vi "CSMLS - Continuous Loop in CSM Example.vi"() -> ()   [LabVIEW 2017]
uses:
  user.lib/_NEVSTOP/Communicable State Machine(CSM)/AdvanceAPI/CSM - Revert Arguments-Safe String.vi
  user.lib/_NEVSTOP/Communicable State Machine(CSM)/AdvanceAPI/CSM - Make String Arguments Safe.vi
  user.lib/_NEVSTOP/Communicable State Machine(CSM)/AdvanceAPI/CSM - Break Down Multiple States String.vi
  user.lib/_NEVSTOP/Communicable State Machine(CSM)/AdvanceAPI/CSM - Compact Multiple States.vi
  user.lib/_NEVSTOP/Communicable State Machine(CSM)/AdvanceAPI/CSM - Keywords.vi
  user.lib/_NEVSTOP/Communicable State Machine(CSM)/_Polymophic/CSM - Filter Duplicated Lines.vi
  user.lib/_NEVSTOP/Communicable State Machine(CSM)/_Shared/Trim Single-line Text.vi
  user.lib/_NEVSTOP/Communicable State Machine(CSM)/Communicable State Machine.lvlib
  user.lib/_NEVSTOP/Communicable State Machine(CSM)/addons/Loop-Support/CSM Loop Support.lvlib
  user.lib/_NEVSTOP/Communicable State Machine(CSM)/addons/Logger/CSM File Logger.lvlib
panel:
  in  "Enable Periodic State Filter(T)":bool=TRUE
  in  "High-Priority Error":bool
  in  "Low-Priority Error":bool
  out "Filtered UI States":string="Macro: DAQ Continuous"
  out "UI States":string="Macro: DAQ Continuous"
  out ">> From CSM >>":string="<loop>"
  out "Remaining States":string="Exit"
  in  "DAQ: Once":bool
  out "Waveform Chart":dbl(graph)=0.33666580363788867
  in  "Center":dbl(slide) scale=0.0..10.0
  in  "Stop":bool
  in  "Start":bool
  out "State History":string="--------------------\nPeroid State:\nFilter #17 since 00:04:42.203 - DAQ: Continuous Check >> 0.902887\rFilter #18 since 00:04:42.203 - Data: Acquisite\n--------------------\n[00:04:45.825] Exit\r[00:04:45.823] Data: Cleanup\r[00:04:45.823] Macro: Exit\r[00:04:45.818] UI: Refresh Buttons <- <end>\r[00:04:45.817] DAQ: Close\r[00:04:45.817] DAQ: Stop\r[00:04:42.203] <Start Filter>DAQ: Continuous Check\r[00:04:42.203] <Start Filter>Data: Acquisite\r[00:04:42.003] DAQ: Continuous Check >> 0.591368 <- <loop>\r[00:04:42.003] Data: Acquisite\r[00:04:41.804] DAQ: Continuous Check >> 0.572752 <- <loop>\r[00:04:41.803] Data: Acquisite\r[00:04:41.603] DAQ: Continuous Check >> 0.632503 <- <loop>\r[00:04:41.603] Data: Acquisite\r[00:04:41.403] DAQ: Continuous Check >> 0.461989 <- <loop>\r[00:04:41.402] Data: Acquisite\r[00:04:41.202] DAQ: Continuous Check <- <loop>\r[00:04:41.201] Data: Acquisite\r[00:04:41.069] UI: Refresh Buttons\r[00:04:41.069] DAQ: Start\r[00:04:41.069] DAQ: Configure\r[00:04:41.069] DAQ: Initialize\r[00:04:41.068] Macro: DAQ Continuous\r[00:04:40.593] Data: Update Indicators\r[00:04:40.588] UI: Refresh Buttons\r[00:04:40.585] UI: Initialize\r[00:04:40.584] Initialize Core Data\r[00:04:40.584] Data: Initialize\r[00:04:40.583] Macro: Initialize\r"
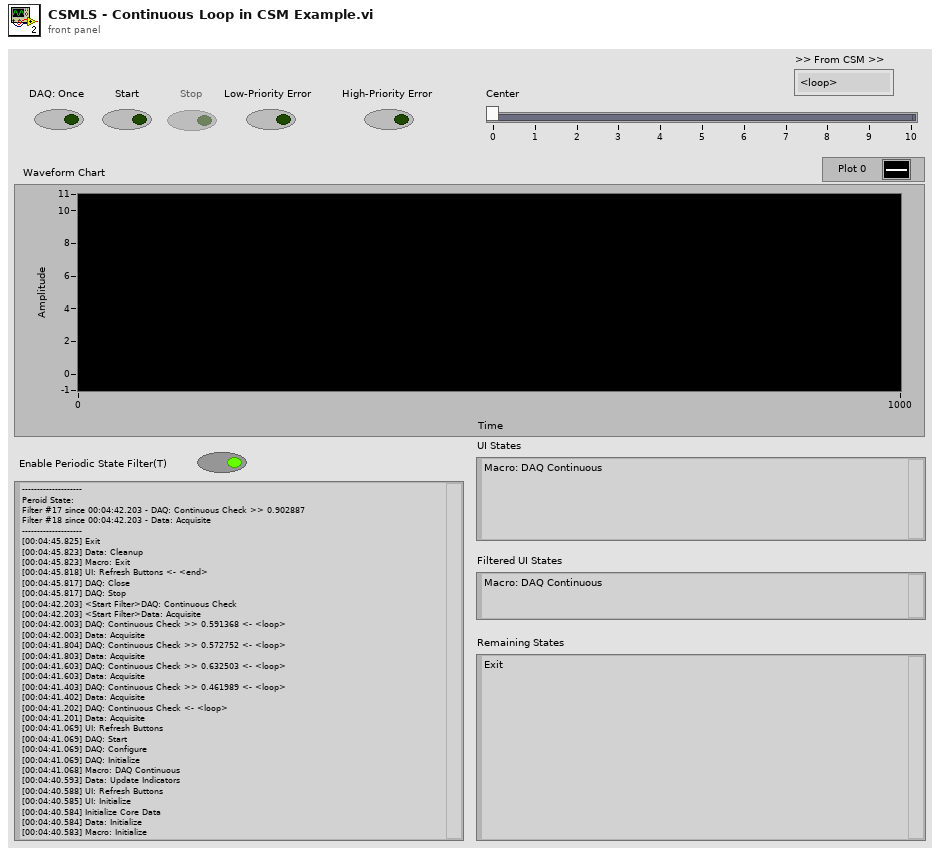
[diagram p1: front panel]
types:
  T1 = enum32{"Invalid", "Standard", "Closed", "Hidden", "Minimized", "Maximized"}
  T2 = enum32{"invalid app kind", "Development System", "Run Time System", "Student Edition", "Embedded LabVIEW", "Evaluation", "Custom"}
  T3 = typedef "Communicable State Machine.lvlib/_CSM_Response Source Message.ctl" = cluster{"‘State":string, "’Arguments":string, "’Error":errorcluster}
  T4 = cluster{"Current VI Reference":refnum<vi>, "Close Panel on Exit?":bool}
  T5 = cluster{"Core":cluster{"Current VI Reference":refnum<vi>, "Close Panel on Exit?":bool}, "IsRunning?":bool, "Center":dbl}
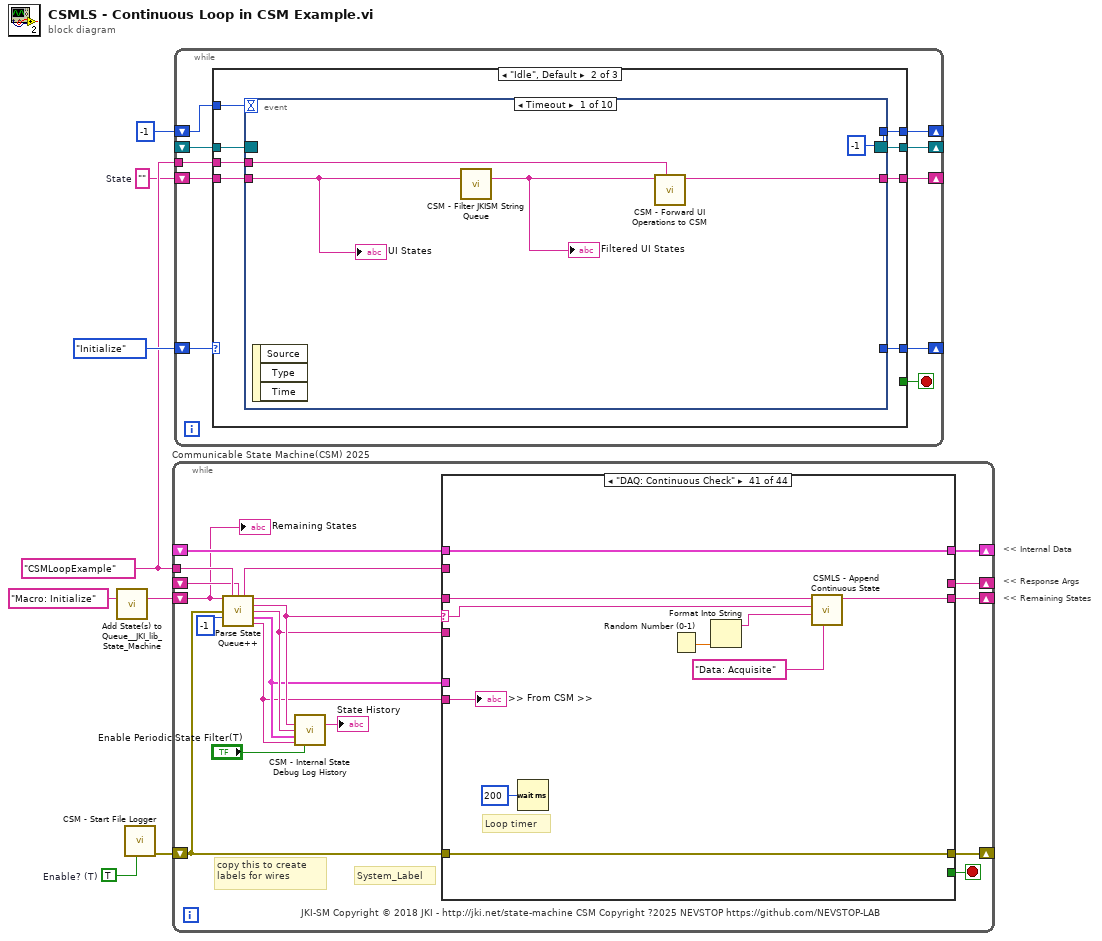
[diagram p0: block diagram]
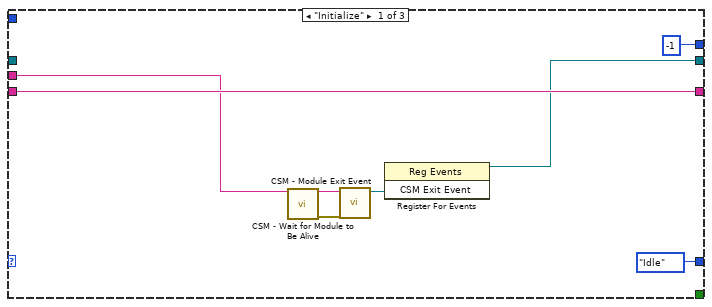
[diagram p2: hidden frame]
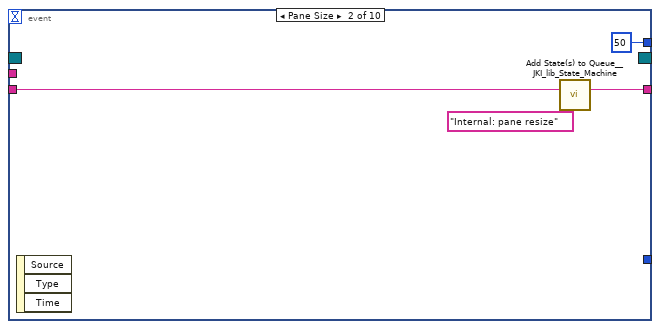
[diagram p3: hidden frame]
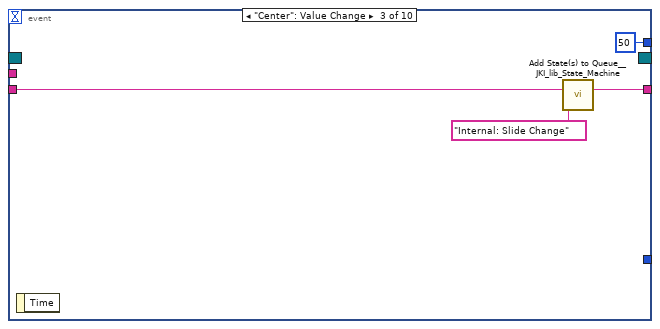
[diagram p4: hidden frame]
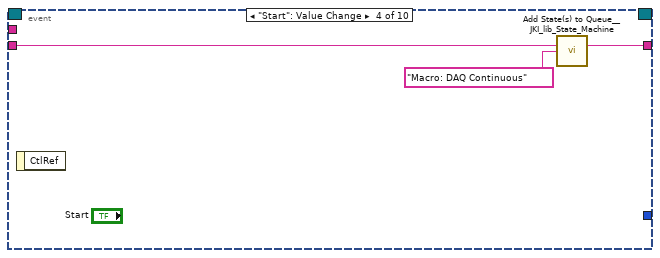
[diagram p5: hidden frame]
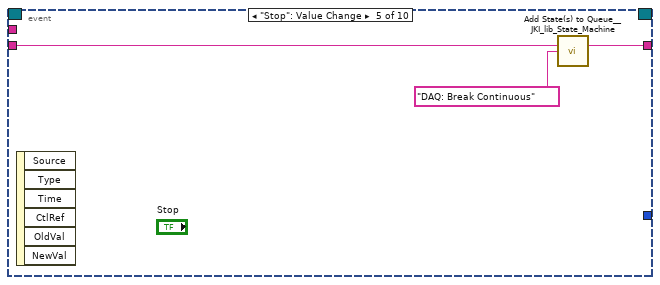
[diagram p6: hidden frame]
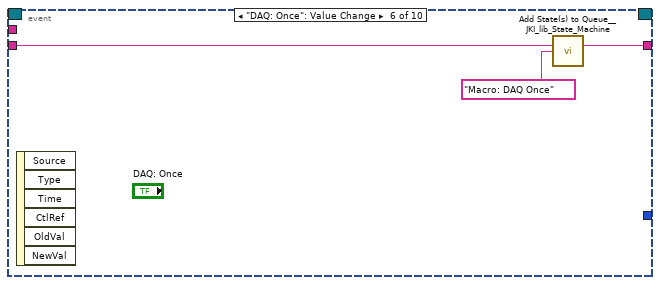
[diagram p7: hidden frame]
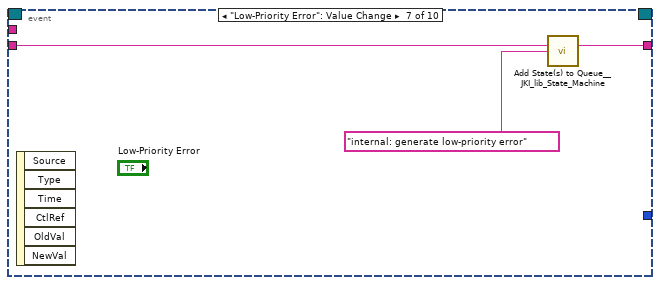
[diagram p8: hidden frame]
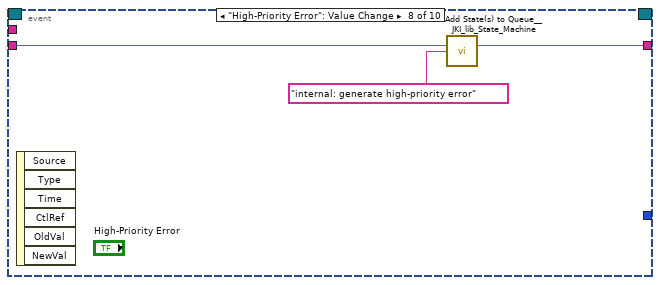
[diagram p9: hidden frame]
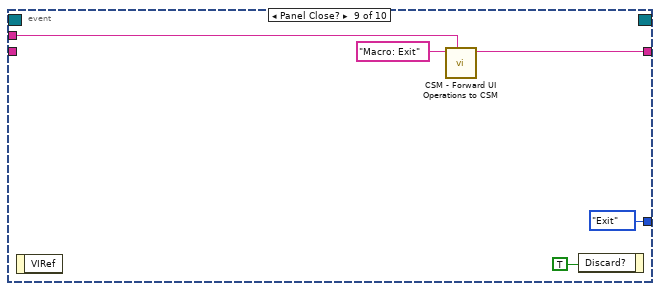
[diagram p10: hidden frame]
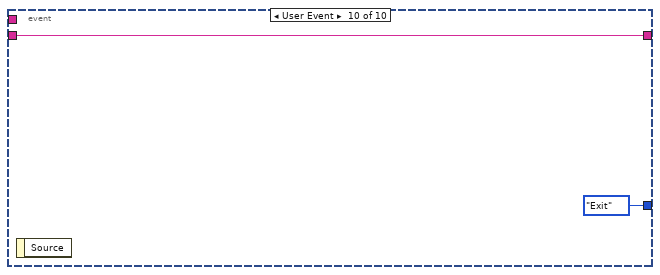
[diagram p11: hidden frame]
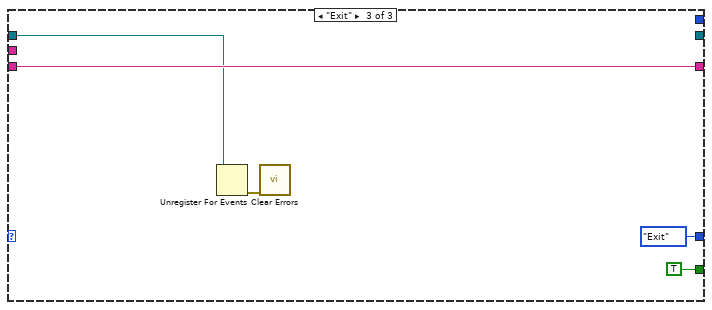
[diagram p12: hidden frame]
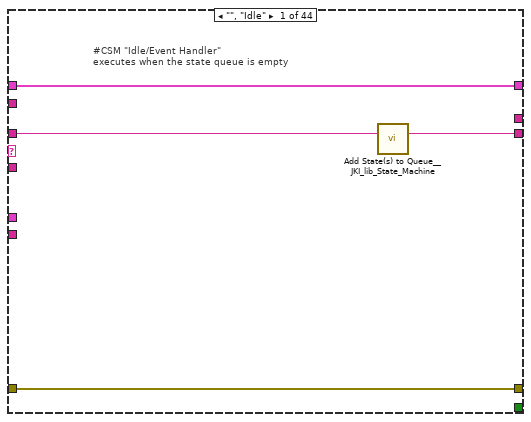
[diagram p13: hidden frame]
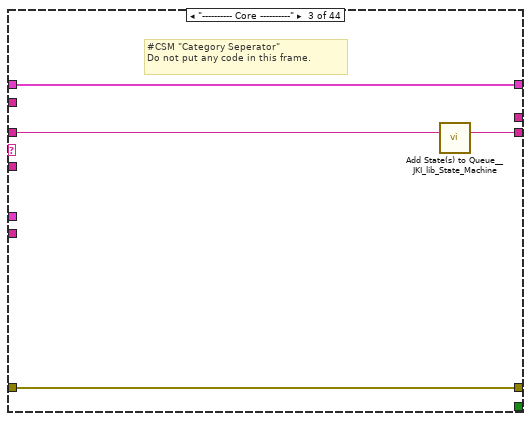
[diagram p15: hidden frame]
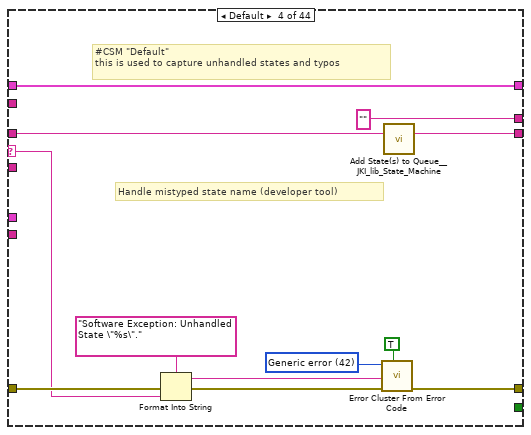
[diagram p16: hidden frame]
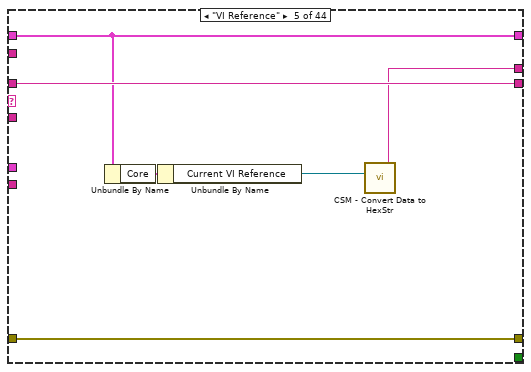
[diagram p17: hidden frame]
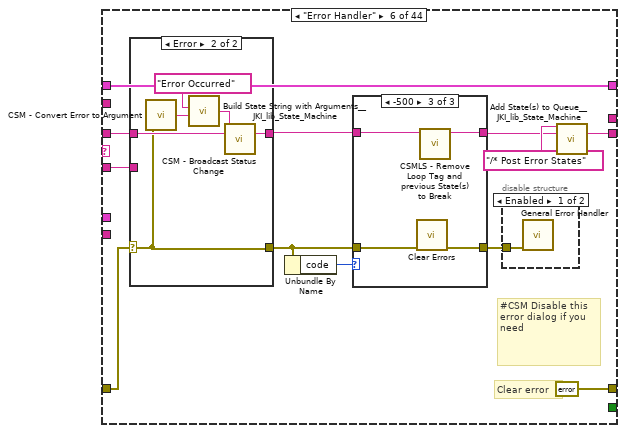
[diagram p18: hidden frame]
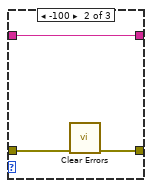
[diagram p20: hidden frame]
diagram:
  w5 = "CSMLoopExample" ("Name (\"\" to Use UUID)")
  w2 = TRUE  # Enable? (T)
  w4 = ""  # State
  # "<< Internal Data"
  # "<< Response Args"
  # "<< Remaining States"
  n1 = call <vilib>:"Add State(s) to Queue__JKI_lib_State_Machine.vi"("State(s) in (\"\")"="Macro: Initialize" ("Init State(\"Macro: Initialize\")")) -> ("States Out"=w7:string)  [unwired: 14 in]
  n2 = call "CSM - Start File Logger.vi"("Enable? (T)"=w2) -> ("error out"=w1:errorcluster)  [unwired: 8 in, 2 out]
  n3 = while "Communicable State Machine(CSM) 2025" {
    shift-right: [w23] -> _
    shift-left: _ -> [w22]
    shift-right: [w26] -> _
    shift-left: w1 -> [w21]
    shift-right: [w25] -> _
    shift-left: w7 -> [w11]
    tunnel: w5 -> [w19]
    shift-right: [w20] -> _
    shift-left: _ -> [w13]
    stop <- w24 stop-if-true
    # "copy this to create labels for wires"
    # "System_Label"
    # "JKI-SM Copyright © 2018 JKI - http://jki.net/state-machine CSM Copyright ?2025 NEVSTOP https://github.com/NEVSTOP-LAB"
    n4 = call "Parse State Queue++.vi"("State Queue"=w11, "Name (\"\" to Use UUID)"=w19, "Response Arguments"=w13, "Previous Error"=w21, "Dequeue (1 ms)"=-1 ("Timeout")) -> ("Name Used"=w14:string, "Remaining States"=w27:string, "Current State"=w18:string, "Arguments"=w17:string, ">> Response Source Message >>"=w16:T3, ">> Source CSM >>"=w15:string)  [unwired: 5 in]
    n5 = call "CSM - Internal State Debug Log History.vi"("State"=w18, "Arguments (\"\")"=w17, ">> Response Source Message >>"=w16, "Source (\"\")"=w15, "Enable Periodic State Filter? (T)"="Enable Periodic State Filter(T)") -> ("Debug Log"=→"State History":string)  [unwired: 10 in]
    n6 = case shown="\"DAQ: Continuous Check\"" w18 {
      selector: w18 -> [_ _ _ w40 _ _ _ w103 _ _ _ _ _ _ _ _ _ _ _ _ _ _ _ _ _ _ _ _ _ _ _ _ _ _ _ _ _ _ _ _ w372 _ _ _]
      tunnel: w27 -> [w28 w33 w38 w44 w55 w65 w97 w105 w115 w126 w140 w145 w149 w156 w158 w165 w169 w175 w181 w196 w274 w279 w284 w286 w291 w297 w309 w313 w318 w325 w329 w333 w337 w341 w344 w346 w349 w352 w357 w364 w374 w380 w386 w389]
      tunnel: w17 -> [_ _ _ _ _ w64 w90 w104 w114 _ _ _ _ _ _ _ _ _ w176 w190 _ _ _ _ _ _ _ _ w316 _ _ _ _ _ _ _ _ _ _ _ _ _ _ _]
      tunnel: w22 -> [w29 w32 w35 w42 w54 w67 w98 w106 w117 w125 w133 w143 w146 _ w157 w160 w166 w173 w179 w192 w273 w276 w281 w288 w293 w299 w308 w312 w317 w322 w326 w330 w336 w340 w343 w345 w348 w351 w356 w366 w377 w381 w385 w388]
      tunnel: [w30 w34 w36 w46 w56 errorcluster {"status"=FALSE, "code"=0, "source"=""} ("error out") w99 w101 w120 w127 w137 w142 w147 w153 w159 w161 w167 w172 w177 w193 w275 w277 w282 w289 w294 w301 w310 w314 w319 w323 w327 w331 w338 errorcluster {"status"=TRUE, "code"=-100, "source"="Low priority error. Daq could continue."} ("error out") errorcluster {"status"=TRUE, "code"=-500, "source"="High priority error. Daq need stop!"} ("error out") w347 w350 w353 w358 w368 w378 w382 w387 w390] -> w26
      tunnel: w21 -> [w30 w34 w36 w45 w56 w66 w99 w108 _ w127 w137 w142 w147 w153 w159 w162 w167 w172 w178 w194 w275 w277 w282 w289 w294 w301 w310 w314 w319 w323 w327 w331 w338 _ _ w347 w350 w353 w358 w368 w378 w382 w387 w390]
      tunnel: [w31 w33 w37 w43 w55 w62 w96 w107 w116 w126 w139 w144 w148 w155 w158 w164 w168 w174 w180 w195 w274 w278 w283 w287 w292 w296 w309 w313 w318 w324 w328 w332 w337 w341 w344 w346 w349 w352 w357 w363 w375 w379 w386 w389] -> w25
      tunnel: [_ _ _ _ _ _ TRUE _ _ _ _ TRUE _ _ _ _ _ _ _ _ _ _ _ _ _ _ _ _ _ _ _ _ _ _ _ _ _ _ _ _ _ _ _ _] -> w24
      tunnel: [w29 w32 w35 w42 w54 w67 w98 w106 w118 w125 w138 w143 w146 w154 w157 w160 w166 w173 w179 w192 w273 w276 w281 w288 w293 w299 w308 w312 w317 w322 w326 w330 w335 w340 w343 w345 w348 w351 w355 w366 w377 w381 w384 w388] -> w23
      tunnel: w15 -> [_ _ _ _ _ _ _ _ w112 _ _ _ _ _ _ _ _ _ _ _ _ _ _ _ _ _ _ _ _ _ _ _ _ _ _ _ _ _ _ _ w373 _ _ _]
      tunnel: w16 -> [_ _ _ _ _ _ _ _ w119 _ _ _ _ _ _ _ _ _ _ _ _ _ _ _ _ _ _ _ _ _ _ _ _ _ _ _ _ _ _ _ _ _ _ _]
      tunnel: [_ _ _ "" w51 _ _ _ _ _ _ _ _ _ _ _ _ _ _ _ _ _ _ _ _ _ _ "API1 Response" w315 _ _ _ _ _ _ _ _ _ _ _ _ _ _ _] -> w20
      tunnel: w14 -> [_ _ _ _ _ _ _ _ _ _ _ _ _ _ _ _ _ _ _ _ _ _ _ _ _ _ _ _ _ _ _ _ _ _ _ _ _ _ _ _ _ _ _ _]
      frame "", "Idle" {
        # "#CSM \"Idle/Event Handler\"\nexecutes when the state queue is empty"
        n7 = call <vilib>:"Add State(s) to Queue__JKI_lib_State_Machine.vi"("State(s) in (\"\")"=w28) -> ("States Out"=w31:string)  [unwired: 14 in]
      }
      frame "CSM Documentation" {
        # "#CSM README FIRST\n\nCSM is a LabVIEW application framework that builds upon JKI State Machine (JKISM). It follows the pattern of JKISM and extends the keywords to describe message communication between CSM modules, including concepts such as Sync-Message, Async-Message, Subscription/Unsubscription of status - essential elements for creating reusable code modules. For more information, please visit the CSM wiki: https://github.com/NEVSTOP-LAB/JKI-State-Machine-Plus-Plus/wiki\n\nFor instructions on JKI State Machine, visit: http://jki.net/state-machine/\nFor information about CSM, visit: https://github.com/NEVSTOP-LAB"
        # "#CSM \"Documentation\"\nCase for holding CSM Documenation"
      }
      frame "---------- Core ----------" {
        # "#CSM \"Category Seperator\"\nDo not put any code in this frame."
        n8 = call <vilib>:"Add State(s) to Queue__JKI_lib_State_Machine.vi"("State(s) in (\"\")"=w38) -> ("States Out"=w37:string)  [unwired: 14 in]
      }
      frame Default {
        w49 = 42 items=["No error", "Argument error", "Memory is full", "Out of zone", "End of file", "File already open", "Generic file I/O error", "File not found", "File permission error", "Disk is full", "Duplicate path", "Too many files open", "System feature not enabled", "Resource file not found", "Cannot add resource", "Resource not found", "Image not found", "Image memory error", "Pen does not exist", "Config type invalid", "Config token not found", "Config parse error", "Config memory error", "Bad external code format", "Bad external code offset", "External code not present", "Null window", "Destroy window error", "Null menu", "Print aborted", "Bad print record", "Print driver error", "Windows error during printing", "Memory error during printing", "Print dialog error", "Generic print error", "Invalid device refnum", "Device not found", "Device parameter error", "Device unit error", "Cannot open device", "Device call aborted", "Generic error", "Cancelled by user", "Object ID too low", "Object ID too high", "Object not in heap", "Unknown heap", "Unknown object (invalid DefProc)", "Unknown object (DefProc not in table)", "Message out of range", "Invalid (null) method", "Unknown message", "Manager call not supported", "Bad address", "Network operation in progress", "Network operation timed out", "Connection is busy", "Network attribute not supported", "Network error", "Address in use", "System out of memory", "Connection aborted", "Connection refused", "Not connected", "Already connected", "Connection closed", "Initialization error (interapplication manager)", "Bad occurrence", "Wait on unbound occurrence handler", "Occurrence queue overflow", "Datalog type conflict", "Unused", "Unrecognized type (interapplication manager)", "Memory corrupt", "Failed to make temporary DLL", "Old CIN version", "Drag socket not found", "Failed to load drop-object", "Failed to register OLE object", "Failed to release OLE object", "Format specifier type mismatch", "Unknown format specifier", "Too few format specifiers", "Too many format specifiers", "Scan failed", "Newer CIN version", "Error converting to variant", "Runtime menu error", "Password tampered", "Variant attribute not found", "Incompatible variant data type", "Event data is not available", "Event Store is not present", "Occurrence is not found", "Event Queue is not created", "Event info is not available", "Refnum passed is NULL", "Error retrieving Class GUID", "Error retrieving CoClass GUID", "Error retrieving TypeLib GUID.", "Bad built application magic bytes.", "Specific driver is different from the specific driver associated with the Logical Name.", "There is no session opened to the class driver.", "Max Error", "MAX - Error with config objects", "MAX - Error loading configuration", "MAX - Group not supported"]
        # "#CSM \"Default\"\nthis is used to capture unhandled states and typos"
        # "Handle mistyped state name (developer tool)"
        n9 = Format Into String(format string="Software Exception: Unhandled State \"%s\"." ("message"), error in=w45, w40) -> (resulting string=w48:string, error out=w47:errorcluster)  [unwired: 1 in]
        n10 = call <vilib>:"Error Cluster From Error Code.vi"("show call chain? (False)"=TRUE, "error in (no error)"=w47, "error message (\"\")"=w48, "error code (0)"=w49) -> ("error out"=w46:errorcluster)  [unwired: 5 in]
        n11 = call <vilib>:"Add State(s) to Queue__JKI_lib_State_Machine.vi"("State(s) in (\"\")"=w44) -> ("States Out"=w43:string)  [unwired: 14 in]
      }
      frame "VI Reference" {
        n12 = Unbundle By Name(w54) -> ("Core"=w53:T4)
        n13 = Unbundle By Name(w53) -> ("Current VI Reference"=w52:refnum<vi>)
        n14 = call "CSM - Convert Data to HexStr.vi"("Variant"=w52) -> ("HEX String (0-9,A-F)"=w51:string)  [unwired: 8 in]
      }
      frame "Error Handler" {
        # "#CSM Disable this error dialog if you need"
        # "Clear error"
        n15 = case shown="Error" w66 {
          selector: w66 -> [_ w83]
          tunnel: [w82 w84] -> w57
          tunnel: w65 -> [w82 w85]
          tunnel: w64 -> [w81 _]
          tunnel: [w80 w83] -> w60
          frame No Error {
            n16 = call "CSM - Convert Argument to Error.vi"("Argument"=w81) -> ("Error"=w80:errorcluster)  [unwired: 4 in]
          }
          frame Error {
            n17 = call "CSM - Convert Error to Argument.vi"("Error"=w83) -> ("Argument"=w87:string)  [unwired: 4 in]
            n18 = call <vilib>:"Build State String with Arguments__JKI_lib_State_Machine.vi"("Arguments (\"\")"=w87, "State"="Error Occurred" ("Status with Arguments")) -> ("State with Arguments"=w86:string)  [unwired: 4 in]
            n19 = call "CSM - Broadcast Status Change.vi"("Status With Arguments"=w86, "State Queue"=w85) -> ("Remaining States"=w84:string)  [unwired: 13 in]
          }
        }
        n20 = Unbundle By Name(w60) -> ("code"=w61:i32)
        n21 = case shown="-500" w61 {
          tunnel: w60 -> [w70 w73 w77]
          tunnel: [w70 w72 w74] -> w59
          tunnel: [w69 w71 w75] -> w58
          tunnel: w57 -> [w69 w71 w76]
          frame 0, Default {
          }
          frame -100 {
            n22 = call <vilib>:"Clear Errors.vi"("error in (no error)"=w73) -> ("error out"=w72:errorcluster)  [unwired: 5 in, 1 out]
          }
          frame -500 {
            n23 = call <vilib>:"Clear Errors.vi"("error in (no error)"=w77) -> ("error out"=w74:errorcluster)  [unwired: 5 in, 1 out]
            n24 = call "CSMLS - Remove Loop Tag and previous State(s) to Break.vi"("States Queue"=w76) -> ("Remaining States"=w75:string)  [unwired: 10 in]
          }
        }
        n25 = disable-structure shown="Enabled" {
          disable-tunnel: w59 -> [w78 w79]
          frame Enabled {
            n26 = call <vilib>:"General Error Handler.vi"("error in (no error)"=w78) -> ()  [unwired: 10 in, 5 out]
          }
          frame Disabled {
            n27 = call <vilib>:"Clear Errors.vi"("error in (no error)"=w79) -> ()  [unwired: 5 in, 2 out]
          }
        }
        n28 = call <vilib>:"Add State(s) to Queue__JKI_lib_State_Machine.vi"("State(s) in Front (\"\")"="/* Post Error States", "State(s) in (\"\")"=w58) -> ("States Out"=w62:string)  [unwired: 13 in]
      }
      frame "Critical Error" {
        w94 = 42 items=["No error", "Argument error", "Memory is full", "Out of zone", "End of file", "File already open", "Generic file I/O error", "File not found", "File permission error", "Disk is full", "Duplicate path", "Too many files open", "System feature not enabled", "Resource file not found", "Cannot add resource", "Resource not found", "Image not found", "Image memory error", "Pen does not exist", "Config type invalid", "Config token not found", "Config parse error", "Config memory error", "Bad external code format", "Bad external code offset", "External code not present", "Null window", "Destroy window error", "Null menu", "Print aborted", "Bad print record", "Print driver error", "Windows error during printing", "Memory error during printing", "Print dialog error", "Generic print error", "Invalid device refnum", "Device not found", "Device parameter error", "Device unit error", "Cannot open device", "Device call aborted", "Generic error", "Cancelled by user", "Object ID too low", "Object ID too high", "Object not in heap", "Unknown heap", "Unknown object (invalid DefProc)", "Unknown object (DefProc not in table)", "Message out of range", "Invalid (null) method", "Unknown message", "Manager call not supported", "Bad address", "Network operation in progress", "Network operation timed out", "Connection is busy", "Network attribute not supported", "Network error", "Address in use", "System out of memory", "Connection aborted", "Connection refused", "Not connected", "Already connected", "Connection closed", "Initialization error (interapplication manager)", "Bad occurrence", "Wait on unbound occurrence handler", "Occurrence queue overflow", "Datalog type conflict", "Unused", "Unrecognized type (interapplication manager)", "Memory corrupt", "Failed to make temporary DLL", "Old CIN version", "Drag socket not found", "Failed to load drop-object", "Failed to register OLE object", "Failed to release OLE object", "Format specifier type mismatch", "Unknown format specifier", "Too few format specifiers", "Too many format specifiers", "Scan failed", "Newer CIN version", "Error converting to variant", "Runtime menu error", "Password tampered", "Variant attribute not found", "Incompatible variant data type", "Event data is not available", "Event Store is not present", "Occurrence is not found", "Event Queue is not created", "Event info is not available", "Refnum passed is NULL", "Error retrieving Class GUID", "Error retrieving CoClass GUID", "Error retrieving TypeLib GUID.", "Bad built application magic bytes.", "Specific driver is different from the specific driver associated with the Logical Name.", "There is no session opened to the class driver.", "Max Error", "MAX - Error with config objects", "MAX - Error loading configuration", "MAX - Group not supported"]
        # "#CSM Stop in Critical Error\nWhen Critical Error occurs, Stop the loop immediately. Do NOT change this unless you fully understand the impact."
        # "#CSM \"Critical Error\"\nWhen any un-recoverable error occurs, CSM goes into this case."
        # "Handle mistyped state name (developer tool)"
        n29 = Format Into String(format string="Software Exception: Critical Error\"%s\"." ("message"), w90) -> (resulting string=w93:string, error out=w92:errorcluster)  [unwired: 2 in]
        n30 = call <vilib>:"Error Cluster From Error Code.vi"("show call chain? (False)"=TRUE, "error in (no error)"=w92, "error message (\"\")"=w93, "error code (0)"=w94) -> ()  [unwired: 5 in, 1 out]
        n31 = call <vilib>:"Add State(s) to Queue__JKI_lib_State_Machine.vi"("State(s) in (\"\")"=w97) -> ("States Out"=w96:string)  [unwired: 14 in]
      }
      frame "Target Error", "Target Timeout Error" {
        # "#CSM \"Target Error\"\nWhen This CSM try to communicate with an un-existed CSM, This CSM goes into this case."
        # "#CSM \"Target Timeout Error\"\nWhen This CSM could not get the sync-call response in time, This CSM goes into this case."
        n32 = Format Into String(format string="Software Exception: %s now \"%s\"." ("message"), error in=w108, w103, w104) -> (resulting string=w102:string)  [unwired: 1 in, 1 out]
        n33 = call "Build Error Cluster.vi"("String to Prepend to Source (\"\")"=w102, "Code"=-1 ("code")) -> ("error out"=w101:errorcluster)
        n34 = call <vilib>:"Add State(s) to Queue__JKI_lib_State_Machine.vi"("State(s) in (\"\")"=w105) -> ("States Out"=w107:string)  [unwired: 14 in]
      }
      frame "Async Response", "Response" {
        n35 = Unbundle(w119) -> ("‘State"=w113:string, "’Arguments"=w111:string, "’Error"=w110:errorcluster)
        n36 = case shown="Default" w113 {
          tunnel: [w124] -> w120
          tunnel: w110 -> [w124]
          tunnel: [w123] -> w118
          tunnel: w117 -> [w123]
          tunnel: [w121] -> w116
          tunnel: w115 -> [w122]
          tunnel: w114 -> [_]
          tunnel: w112 -> [_]
          tunnel: w111 -> [_]
          frame Default {
            # "#CSM Response Comments\nAfter Message is executed, CSM goes to this state for receive the response.\n    For Async Message(->), \"Async Response\" is used. This CSM will goes to \"Async Message Posted\" immediately and receive the \"Async Response\" after the callee finishes the message.\n    For Sync Message(@),  This CSM will wait until the message is done and immediately goes to \"Response\""
            # "#CSM \"Async Response\"\nHandle Async-call Response (\"Async Response\" for ->)"
            # "#CSM \"Response\"\nHandle Sync-call Response (\"Response\" for -@)"
            n37 = call <vilib>:"Add State(s) to Queue__JKI_lib_State_Machine.vi"("State(s) in (\"\")"=w122) -> ("States Out"=w121:string)  [unwired: 14 in]
          }
        }
      }
      frame "Async Message Posted" {
        # "#CSM \"Async Message Posted\"\nAfter Async Message is posted (-> or ->| ), CSM goes to this state for post-action.\nYou can use Argument - State to tell which Async Message is called."
      }
      frame "Initialize Core Data" {
        # "#CSM \"Initialize Core Data\"\nThis is used to determine panel behavior on exit"
        # "originally closed?"
        # "exe?"
        # "If panel starts closed or is an EXE, then close it when we exit"
        n38 = property class="VI"() -> ("FP.State"=w130:T1)  [unwired: 2 in, 2 out]
        n39 = property class="App"() -> ("App.Kind"=w136:T2)  [unwired: 2 in, 2 out]
        n40 = control-ref of="Current VI Reference"() -> (w131:refnum<vi>)
        n41 = Equal?(x=w130, y=T1."Closed" ("Front Panel Window:State")) -> (x = y?=w128:bool)
        n42 = Equal?(x=w136, y=T2."Run Time System" ("Application:Kind")) -> (x = y?=w134:bool)
        n43 = Or(x=w128, y=w134) -> (x .or. y?=w132:bool)
        n44 = Bundle By Name(cluster=w133, "Core.Current VI Reference"=w131, "Core.Close Panel on Exit?"=w132) -> (w138:T5)
        n45 = call <vilib>:"Add State(s) to Queue__JKI_lib_State_Machine.vi"("State(s) in (\"\")"=w140) -> ("States Out"=w139:string)  [unwired: 14 in]
      }
      frame "Exit" {
        # "#CSM \"Exit\"\nCase for exiting the loop. No errors that occur here will be handled."
        n46 = call <vilib>:"Add State(s) to Queue__JKI_lib_State_Machine.vi"("State(s) in (\"\")"=w145) -> ("States Out"=w144:string)  [unwired: 14 in]
      }
      frame "---------- Data ----------" {
        # "#CSM \"Category Seperator\"\nDo not put any code in this frame."
        n47 = call <vilib>:"Add State(s) to Queue__JKI_lib_State_Machine.vi"("State(s) in (\"\")"=w149) -> ("States Out"=w148:string)  [unwired: 14 in]
      }
      frame "Data: Initialize" {
        w151 = T4 {"Current VI Reference"=refnum, "Close Panel on Exit?"=FALSE}  # Core
        w152 = FALSE  # IsRunning?
        # "do not delete - used by framework"
        # "Expand Bundle to add new data elements to shift register data."
        # "Initialize the shift-register data, here.\n(data names are defined by what you wire into the bundle function)"
        n48 = local read "Center"() -> (w150:dbl)
        n49 = Bundle("Core"=w151, "IsRunning?"=w152, "Center"=w150) -> (w154:T5)  [unwired: 1 in]
        n50 = call <vilib>:"Add State(s) to Queue__JKI_lib_State_Machine.vi"("State(s) in (\"\")"=w156) -> ("States Out"=w155:string)  [unwired: 14 in]
      }
      frame "Data: Update Indicators" {
      }
      frame "Data: Cleanup" {
        # "Cleanup any data and references, here.\n(this is called automatically, by the Macro: Exit)"
        n51 = Unbundle By Name(w160) -> ("Core.Current VI Reference"=w163:refnum<vi>)
        n52 = Close Reference(reference=w163, error in (no error)=w162) -> (error out=w161:errorcluster)
        n53 = call <vilib>:"Add State(s) to Queue__JKI_lib_State_Machine.vi"("State(s) in (\"\")"=w165) -> ("States Out"=w164:string)  [unwired: 14 in]
      }
      frame "---------- UI ----------" {
        # "#CSM \"Category Seperator\"\nDo not put any code in this frame."
        n54 = call <vilib>:"Add State(s) to Queue__JKI_lib_State_Machine.vi"("State(s) in (\"\")"=w169) -> ("States Out"=w168:string)  [unwired: 14 in]
      }
      frame "UI: Initialize" {
        # "#CSM \"UI: Initialize\"\nInitialize the User Interface, here.\n(this is called automatically, by the Macro: Init)"
        n55 = property on="Waveform Chart" class="WFChart (strict)"("History Data"=dbl[] []) -> ()  [unwired: 2 in, 2 out]
        n56 = call <vilib>:"Add State(s) to Queue__JKI_lib_State_Machine.vi"("State(s) in Front (\"\")"="UI: Refresh Buttons" ("State(s) in Front (\"\")"), "State(s) in (\"\")"=w175) -> ("States Out"=w174:string)  [unwired: 13 in]
      }
      frame "UI: Cursor Set" {
        # "#CSM \"UI: Cursor Set\"\nSet and Unset Cursor Busy.\n(Usage: \"UI: Cursor Set >> Busy|Idle\")"
        # "Argument"
        n57 = disable-structure shown="TARGET_TYPE!=Windows" {
          disable-tunnel: w178 -> [w184 w189]
          disable-tunnel: [w183 w189] -> w177
          disable-tunnel: w176 -> [w182 _]
          frame condition #0 (active) {
            n58 = case shown="\"Idle\", Default" w182 {
              tunnel: w184 -> [w186 w188]
              tunnel: [w185 w187] -> w183
              frame "Idle", Default {
                n59 = call <vilib>:"Unset Busy.vi"("error in (no error)"=w186) -> ("error out"=w185:errorcluster)  [unwired: 10 in]
              }
              frame "Busy" {
                n60 = call <vilib>:"Set Busy.vi"("error in (no error)"=w188) -> ("error out"=w187:errorcluster)  [unwired: 9 in, 1 out]
              }
            }
          }
          frame condition #1 {
          }
        }
        n61 = call <vilib>:"Add State(s) to Queue__JKI_lib_State_Machine.vi"("State(s) in (\"\")"=w181) -> ("States Out"=w180:string)  [unwired: 14 in]
      }
      frame "UI: Front Panel State" {
        # "#CSM \"UI: Front Panel State\"\nSet Front Panel Open or Closed\n(Usage: \"UI: Front Panel State >> Open|Close\")"
        # "Argument"
        n62 = Unbundle By Name(w192) -> ("Core.Current VI Reference"=w191:refnum<vi>)
        n63 = call <vilib>:"Add State(s) to Queue__JKI_lib_State_Machine.vi"("State(s) in (\"\")"=w196) -> ("States Out"=w195:string)  [unwired: 14 in]
        n64 = case shown="\"Close\", \"Closed\"" w190 {
          tunnel: w194 -> [w202 w217 w228 w241 w254]
          tunnel: [w204 w218 w230 w243 w256] -> w193
          tunnel: w191 -> [w203 w215 w229 w242 w255]
          frame "Open", "Standard", Default {
            w197 = T1."Standard" ("State")
            n65 = property class="VI"(reference=w203, error in=w202) -> (reference out=w200:refnum<vi>, error out=w201:errorcluster, "FP.State"=w199:T1)
            n66 = Not Equal?(x=w199, y=w197) -> (x != y?=w198:bool)
            n67 = case shown="True" w198 {
              tunnel: [w208 w210] -> w204
              tunnel: w201 -> [w207 w210]
              tunnel: w200 -> [w206 _]
              tunnel: w197 -> [w205 _]
              frame True {
                n68 = invoke class="VI" method="FP.Open"(reference=w206, error in=w207, "Activate"=TRUE, "State"=w205) -> (error out=w208:errorcluster)  [unwired: 1 in, 4 out]
              }
              frame False {
              }
            }
          }
          frame "Close", "Closed" {
            n69 = property class="VI"(reference=w215, error in=w217) -> (reference out=w214:refnum<vi>, error out=w216:errorcluster, "FP.State"=w212:T1)
            n70 = Not Equal?(x=w212, y=T1."Closed" ("Front Panel Window:State")) -> (x != y?=w211:bool)
            n71 = case shown="False" w211 {
              tunnel: [w219 w222] -> w218
              tunnel: w216 -> [w219 w221]
              tunnel: w214 -> [_ w220]
              frame False {
              }
              frame True {
                n72 = invoke class="VI" method="FP.Close"(reference=w220, error in=w221) -> (error out=w222:errorcluster)  [unwired: 1 in, 2 out]
              }
            }
          }
          frame "Hidden", "Hide" {
            w223 = T1."Hidden" ("State")
            n73 = property class="VI"(reference=w229, error in=w228) -> (reference out=w226:refnum<vi>, error out=w227:errorcluster, "FP.State"=w225:T1)
            n74 = Not Equal?(x=w225, y=w223) -> (x != y?=w224:bool)
            n75 = case shown="True" w224 {
              tunnel: [w234 w235] -> w230
              tunnel: w227 -> [w233 w235]
              tunnel: w226 -> [w232 _]
              tunnel: w223 -> [w231 _]
              frame True {
                n76 = invoke class="VI" method="FP.Open"(reference=w232, error in=w233, "State"=w231) -> (error out=w234:errorcluster)  [unwired: 2 in, 4 out]
              }
              frame False {
              }
            }
          }
          frame "Minimize", "Minimized" {
            w236 = T1."Minimized" ("State")
            n77 = property class="VI"(reference=w242, error in=w241) -> (reference out=w239:refnum<vi>, error out=w240:errorcluster, "FP.State"=w238:T1)
            n78 = Not Equal?(x=w238, y=w236) -> (x != y?=w237:bool)
            n79 = case shown="True" w237 {
              tunnel: [w247 w248] -> w243
              tunnel: w240 -> [w246 w248]
              tunnel: w239 -> [w245 _]
              tunnel: w236 -> [w244 _]
              frame True {
                n80 = invoke class="VI" method="FP.Open"(reference=w245, error in=w246, "State"=w244) -> (error out=w247:errorcluster)  [unwired: 2 in, 4 out]
              }
              frame False {
              }
            }
          }
          frame "Maximize", "Maximized" {
            w249 = T1."Maximized" ("State")
            n81 = property class="VI"(reference=w255, error in=w254) -> (reference out=w252:refnum<vi>, error out=w253:errorcluster, "FP.State"=w251:T1)
            n82 = Not Equal?(x=w251, y=w249) -> (x != y?=w250:bool)
            n83 = case shown="True" w250 {
              tunnel: [w260 w261] -> w256
              tunnel: w253 -> [w259 w261]
              tunnel: w252 -> [w258 _]
              tunnel: w249 -> [w257 _]
              frame True {
                n84 = invoke class="VI" method="FP.Open"(reference=w258, error in=w259, "State"=w257) -> (error out=w260:errorcluster)  [unwired: 2 in, 4 out]
              }
              frame False {
              }
            }
          }
        }
      }
      frame "UI: Refresh Buttons" {
        # ":)"
        n85 = Unbundle By Name(w273) -> ("IsRunning?"=w263:bool)
        n86 = control-ref of="DAQ: Once"() -> (w272:refnum<vi>)
        n87 = control-ref of="Stop"() -> (w271:refnum<vi>)
        n88 = control-ref of="Start"() -> (w270:refnum<vi>)
        n89 = Not(x=w263) -> (.not. x?=w262:bool)
        n90 = Boolean To (0,1)(Boolean=w263) -> (0, 1=w269:i16)
        n91 = Boolean To (0,1)(Boolean=w262) -> (0, 1=w266:i16)
        n92 = Multiply(x=i16 2, y=w269) -> (x*y=w268:i16)
        n93 = Multiply(x=i16 2, y=w266) -> (x*y=w264:i16)
        n94 = property class="Bool"(reference=w272, "DisabledEnum"=w268) -> ()  [unwired: 1 in, 2 out]
        n95 = property class="Bool"(reference=w271, "DisabledEnum"=w264) -> ()  [unwired: 1 in, 2 out]
        n96 = property class="Bool"(reference=w270, "DisabledEnum"=w268) -> ()  [unwired: 1 in, 2 out]
      }
      frame "---------- Macro ----------" {
        # "#CSM \"Category Seperator\"\nDo not put any code in this frame."
        n97 = call <vilib>:"Add State(s) to Queue__JKI_lib_State_Machine.vi"("State(s) in (\"\")"=w279) -> ("States Out"=w278:string)  [unwired: 14 in]
      }
      frame "Macro: Initialize" {
        # "#CSM \"Macro: Initialize\"\nInitialization Macro (This is called once, when the VI starts)"
        n98 = call <vilib>:"Add State(s) to Queue__JKI_lib_State_Machine.vi"("State(s) in Front (\"\")"="Data: Initialize\nInitialize Core Data\nUI: Initialize\nData: Update Indicators", "State(s) in (\"\")"=w284) -> ("States Out"=w283:string)  [unwired: 13 in]
      }
      frame "Macro: DAQ Once" {
        n99 = call <vilib>:"Add State(s) to Queue__JKI_lib_State_Machine.vi"("State(s) in Front (\"\")"="DAQ: Initialize\nDAQ: Configure\nDAQ: Start\nData: Acquisite\nDAQ: Stop\nDAQ: Close\nUI: Refresh Buttons" ("State(s) in Front (\"\")"), "State(s) in (\"\")"=w286) -> ("States Out"=w287:string)  [unwired: 13 in]
      }
      frame "Macro: DAQ Continuous" {
        n100 = call "CSMLS - Define Loop State(s).vi"("Loop State (S) And Arguments"="DAQ: Initialize \nDAQ: Configure\nDAQ: Start\nUI: Refresh Buttons\nData: Acquisite\nDAQ: Continuous Check -><loop> \nDAQ: Stop\nDAQ: Close \nUI: Refresh Buttons" ("State(s) in Front (\"\")"), "States Queue"=w291) -> ("Remaining States"=w292:string)  [unwired: 13 in]
      }
      frame "Macro: Exit" {
        # "#github 288\nhttps://github.com/NEVSTOP-LAB/Communicable-State-Machine/issues/288\nNo need to call CSMLS - Add Exit State(s) with Loop Check.vi. Parse State Queue++.vi will handle it. \nLoop will be stopped before entering \"Macro: Exit\" state by remove -><loop> and previous states in Parse State Queue++.vi."
        # "#CSM \"Macro: Exit\"\nExit Macro (This is called once, when the VI exits)"
        n101 = call <vilib>:"Add State(s) to Queue__JKI_lib_State_Machine.vi"("State(s) in (\"\")"="//Exit Sub-Modules ", "State(s) at Back (\"\")"="Data: Cleanup\nExit") -> ("States Out"=w295:string)  [unwired: 13 in]
        n102 = disable-structure shown="Enabled" {
          disable-tunnel: w297 -> [w304 w306]
          disable-tunnel: [w303 w307] -> w296
          disable-tunnel: w295 -> [w302 w305]
          frame Disabled {
            n103 = call "CSMLS - Add Exit State(s) with Loop Check.vi"("Exiting States"=w302, "States Queue"=w304) -> ("Remaining States"=w303:string)  [unwired: 12 in, 1 out]
          }
          frame Enabled {
            n104 = call <vilib>:"Add State(s) to Queue__jki_lib_state_machine.vi"("State(s) in Front (\"\")"=w305, "State(s) in (\"\")"=w306) -> ("States Out"=w307:string)  [unwired: 13 in]
          }
        }
      }
      frame "---------- API ----------" {
        # "#CSM \"Category Seperator\"\nDo not put any code in this frame."
      }
      frame "API: API1" {
        # "#CSM API Example\nCopy/Rename this case for your own API"
        # "#CSM Response\nConnect this to return the response of your API"
        # "#CSM >> From CSM >>\nIf you need to tell who triggered this state , use this string. If it's this case itself, this string is \"\"."
        # "#CSM >> Arguments >>\nDeal with the parameter if any"
      }
      frame "API: API2" {
        # "#CSM API Example\nCopy/Rename this case for your own API"
        # "unpack Hex String  to Variant\nif complex parameter is needed."
        n105 = call "CSM - Convert HexStr to Data.vi"("HEX String"=w316) -> ()  [unwired: 7 in, 2 out]
        n106 = disable-structure shown="Disabled" {
          disable-tunnel: [w320 "API2 Response"] -> w315
          frame Disabled {
            # "pack variant to hexstr \nif complex response is needed."
            # "complex Response"
            n107 = call "CSM - Convert Data to HexStr.vi"() -> ("HEX String (0-9,A-F)"=w320:string)  [unwired: 9 in]
          }
          frame Enabled {
          }
        }
      }
      frame "---------- Internal ----------" {
        # "#CSM \"Category Seperator\"\nDo not put any code in this frame."
        n108 = call <vilib>:"Add State(s) to Queue__JKI_lib_State_Machine.vi"("State(s) in (\"\")"=w325) -> ("States Out"=w324:string)  [unwired: 14 in]
      }
      frame "Internal: button click" {
        # "#CSM \"Internal State\"\nThis category is used for holding internal states"
        n109 = call <vilib>:"Add State(s) to Queue__JKI_lib_State_Machine.vi"("State(s) in (\"\")"=w329) -> ("States Out"=w328:string)  [unwired: 14 in]
      }
      frame "Internal: pane resize" {
        # "#CSM \"Internal State\"\nThis category is used for holding internal states"
        n110 = call <vilib>:"Add State(s) to Queue__JKI_lib_State_Machine.vi"("State(s) in (\"\")"=w333) -> ("States Out"=w332:string)  [unwired: 14 in]
      }
      frame "Internal: Slide Change" {
        n111 = Bundle By Name(cluster=w336, "Center"="Center") -> (w335:T5)
      }
      frame "internal: generate low-priority error" {
      }
      frame "internal: generate high-priority error" {
      }
      frame "----------- daq ---------------" {
      }
      frame "DAQ: Initialize" {
      }
      frame "DAQ: Configure" {
      }
      frame "DAQ: Start" {
        n112 = Bundle By Name(cluster=w356, "IsRunning?"=TRUE) -> (w355:T5)
      }
      frame "Data: Acquisite" {
        n113 = Unbundle By Name(w366) -> ("Center"=w365:dbl)
        n114 = Random Number (0-1)() -> (number: 0 to 1=w367:dbl)
        n115 = Add(x=w367, y=w365) -> (x+y=w360:dbl)
        "Waveform Chart" <- w360
        n116 = Format Into String(w360) -> (resulting string=w359:string)  [unwired: 3 in, 1 out]
        n117 = call <vilib>:"Build State String with Arguments__JKI_lib_State_Machine.vi"("Arguments (\"\")"=w359, "State"="Data") -> ("State with Arguments"=w362:string)  [unwired: 4 in]
        n118 = call "CSM - Broadcast Status Change.vi"("Status With Arguments"=w362, "State Queue"=w364) -> ("Remaining States"=w363:string)  [unwired: 13 in]
      }
      frame "DAQ: Continuous Check" {
        # "Loop timer"
        n119 = Wait (ms)(milliseconds to wait=u32 200) -> ()  [unwired: 1 out]
        n120 = Random Number (0-1)() -> (number: 0 to 1=w370:dbl)
        n121 = Format Into String(w370) -> (resulting string=w369:string)  [unwired: 3 in, 1 out]
        n122 = call "CSMLS - Append Continuous State.vi"("Loop State (S) And Arguments"="Data: Acquisite" ("Loop State(s) and Arguments"), "Continous Arguments (\"\")"=w369, "Continous State"=w372, "States Queue"=w374) -> ("Remaining States"=w375:string)  [unwired: 7 in]
        ">> From CSM >>" <- w373
      }
      frame "DAQ: Break Continuous" {
        n123 = call "CSMLS - Remove Loop Tag to Break.vi"("States Queue"=w380) -> ("Remaining States"=w379:string)  [unwired: 10 in]
      }
      frame "DAQ: Stop" {
        n124 = Bundle By Name(cluster=w385, "IsRunning?"=FALSE) -> (w384:T5)
      }
      frame "DAQ: Close" {
      }
    }
    "Remaining States" <- w11
  }
  n125 = while {
    shift-right: [w399] -> _
    shift-left: enum16{"Idle", "Initialize", "Exit"}."Initialize" -> [w400]
    tunnel: w5 -> [w397]
    shift-right: [w395] -> _
    shift-left: w4 -> [w396]
    shift-right: [w393] -> _
    shift-left: -1 -> [w394]
    shift-right: [w392] -> _
    shift-left: _ -> [w391]
    stop <- w398 stop-if-true
    n126 = case shown="\"Idle\", Default" w400 {
      tunnel: [enum16{"Idle", "Initialize", "Exit"}."Idle" w416 enum16{"Idle", "Initialize", "Exit"}."Exit"] -> w399
      tunnel: [_ _ TRUE] -> w398
      tunnel: w397 -> [w404 w415 _]
      tunnel: w396 -> [w407 w413 w454]
      tunnel: [w407 w414 w454] -> w395
      tunnel: w394 -> [_ w411 _]
      tunnel: [-1 w412 _] -> w393
      tunnel: [w403 w409 _] -> w392
      tunnel: w391 -> [_ w410 w453]
      frame "Initialize" {
        n127 = call "CSM - Wait for Module to Be Alive.vi"("CSM Name"=w404) -> ("CSM Name (Dup)"=w402:string, "error out"=w401:errorcluster)  [unwired: 12 in, 1 out]
        n128 = call "CSM - Module Exit Event.vi"("Error In"=w401, "Name (\"\" to Use UUID) In"=w402) -> ("CSM Exit Event"=w405:refnum<user-event>)  [unwired: 7 in, 2 out]
        n129 = register-events(w405) -> (reference out=w403:refnum<event-registration>)  [unwired: 2 in, 1 out]
      }
      frame "Idle", Default {
        n130 = event shown="[0] Timeout" {
          selector: w410 -> [_ _ _ _ _ _ _ _ _ _]
          dyn-events: [_ _ _ _ _ _ _ _ _ _] -> w409
          timeout: w411 -> [_ _ _ _ _ _ _ _ _ _]
          tunnel: [_ _ _ _ _ _ _ _ enum16{"Idle", "Initialize", "Exit"}."Exit" enum16{"Idle", "Initialize", "Exit"}."Exit"] -> w416
          tunnel: w415 -> [w419 _ _ _ _ _ _ _ w446 _]
          tunnel: w413 -> [w417 w425 w429 w432 w434 w437 w441 w443 _ w451]
          tunnel: [w420 w424 w428 w431 w435 w438 w440 w442 w445 w451] -> w414
          tunnel: [-1 50 50 _ _ _ _ _ _ _] -> w412
          event Timeout {
            n131 = event-data() -> ()  [unwired: 1 in, 3 out]
            n132 = call-poly "CSM - Filter JKISM String Queue.vi"("State (S) In (\"\")"=w417) -> ("States Out"=w418:string)  [unwired: 14 in]
            "Filtered UI States" <- w418
            n133 = call "CSM - Forward UI Operations to CSM.vi"("Name (\"\" to Use UUID)"=w419, "State (S) In (\"\")"=w418) -> ("States Out"=w420:string)  [unwired: 9 in]
            "UI States" <- w417
          }
          event Pane Size {
            n134 = event-data() -> ()  [unwired: 1 in, 3 out]
            n135 = call <vilib>:"Add State(s) to Queue__JKI_lib_State_Machine.vi"("State(s) in (\"\")"=w425, "State(s) at Back (\"\")"="Internal: pane resize" ("State(s) at Back (\"\")")) -> ("States Out"=w424:string)  [unwired: 13 in]
          }
          event "Center": Value Change {
            n136 = event-data() -> ()  [unwired: 1 in, 1 out]
            n137 = call <vilib>:"Add State(s) to Queue__JKI_lib_State_Machine.vi"("State(s) in (\"\")"=w429, "State(s) at Back (\"\")"="Internal: Slide Change" ("State(s) at Back (\"\")")) -> ("States Out"=w428:string)  [unwired: 13 in]
          }
          event "Start": Value Change {
            n138 = event-data() -> ()  [unwired: 1 in, 1 out]
            n139 = call <vilib>:"Add State(s) to Queue__JKI_lib_State_Machine.vi"("State(s) in (\"\")"=w432, "State(s) at Back (\"\")"="Macro: DAQ Continuous" ("State(s) at Back (\"\")")) -> ("States Out"=w431:string)  [unwired: 13 in]
          }
          event "Stop": Value Change {
            n140 = event-data() -> ()  [unwired: 1 in, 6 out]
            n141 = call <vilib>:"Add State(s) to Queue__JKI_lib_State_Machine.vi"("State(s) in (\"\")"=w434, "State(s) at Back (\"\")"="DAQ: Break Continuous" ("State(s) at Back (\"\")")) -> ("States Out"=w435:string)  [unwired: 13 in]
          }
          event "DAQ: Once": Value Change {
            n142 = event-data() -> ()  [unwired: 1 in, 6 out]
            n143 = call <vilib>:"Add State(s) to Queue__JKI_lib_State_Machine.vi"("State(s) in (\"\")"=w437, "State(s) at Back (\"\")"="Macro: DAQ Once" ("State(s) at Back (\"\")")) -> ("States Out"=w438:string)  [unwired: 13 in]
          }
          event "Low-Priority Error": Value Change {
            n144 = event-data() -> ()  [unwired: 1 in, 6 out]
            n145 = call <vilib>:"Add State(s) to Queue__JKI_lib_State_Machine.vi"("State(s) in (\"\")"=w441, "State(s) at Back (\"\")"="internal: generate low-priority error" ("State(s) at Back (\"\")")) -> ("States Out"=w440:string)  [unwired: 13 in]
          }
          event "High-Priority Error": Value Change {
            n146 = event-data() -> ()  [unwired: 1 in, 6 out]
            n147 = call <vilib>:"Add State(s) to Queue__JKI_lib_State_Machine.vi"("State(s) in (\"\")"=w443, "State(s) at Back (\"\")"="internal: generate high-priority error" ("State(s) at Back (\"\")")) -> ("States Out"=w442:string)  [unwired: 13 in]
          }
          event Panel Close? {
            n148 = event-data() -> ()  [unwired: 1 in, 1 out]
            n149 = call "CSM - Forward UI Operations to CSM.vi"("Name (\"\" to Use UUID)"=w446, "State (S) In (\"\")"="Macro: Exit" ("State")) -> ("States Out"=w445:string)  [unwired: 9 in]
            n150 = event-data("Discard?"=TRUE) -> ()  [unwired: 1 in, 1 out]
          }
          event User Event {
            n151 = event-data() -> ()  [unwired: 1 in, 1 out]
          }
        }
      }
      frame "Exit" {
        n152 = Unregister For Events(event registration refnum=w453) -> (error out=w452:errorcluster)  [unwired: 1 in]
        n153 = call <vilib>:"Clear Errors.vi"("error in (no error)"=w452) -> ()  [unwired: 5 in, 2 out]
      }
    }
  }
